vi "ex8-2.vi"   [LabVIEW 2009]
uses:
  <vilib>/NXT/Remote Library/Sound/NXT_SoundVolume.ctl
  <vilib>/NXT/Dual Mode Library/Waits/Wait_Num.vi
  <vilib>/NXT/Dual Mode Library/Sound/PlaySoundFile.vi
types:
  T1 = typedef "NXT_SoundVolume.ctl" = u8
  T2 = typedef "LVHSConnector.ctl" = cluster{"error":errorcluster, "address":string, "NXT #":i32, "Show Error":bool, "Connection":u16}
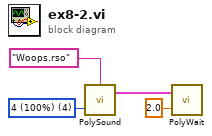
[diagram p0: block diagram]
diagram:
  w3 = T1 4 items=["0 (Mute)", "1 (25%)", "2 (50%)", "3 (75%)", "4 (100%)"] ("Volume (4)")
  n1 = call-poly <vilib>:"PolySound.vi"("Volume (4)"=w3, "Filename (*.rso)"="Woops.rso") -> ("NXT"=w1:T2)  [unwired: 2 in]
  n2 = call-poly <vilib>:"PolyWait.vi"("Time (1 sec)"=sgl 2.0, "NXT"=w1) -> ()  [unwired: 2 in, 1 out]
